vi "sv_UFF58 Get Channel Name.vi"(0 "channel name":string) -> (4 "numerator channel name":string, 6 "denominator channel name":string)   [LabVIEW 2017, in "SoundVib_UFF58.lvlib"]
doc: "This VI extracts <B>numerator channel name</B> and <B>denominator channel name</B> from <B>channel name</B>. It is used mainly when we want to get the channel name from the spectrum info."
uses:
  <vilib>/addons/Sound and Vibration/svt_UFF58/SoundVib_UFF58.lvlib
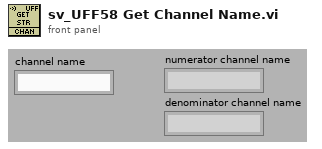
[diagram p1: front panel]
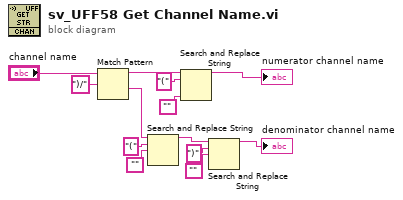
[diagram p0: block diagram]
diagram:
  n1 = Match Pattern(string="channel name", regular expression=")/") -> (before substring=w10:string, after substring=w6:string)  [unwired: 1 in, 2 out]
  n2 = Search and Replace String(input string=w6, search string="(", replace string="") -> (result string=w9:string)  [unwired: 5 in, 3 out]
  n3 = Search and Replace String(input string=w10, search string="(", replace string="") -> (result string=→"numerator channel name":string)  [unwired: 5 in, 3 out]
  n4 = Search and Replace String(input string=w9, search string=")", replace string="") -> (result string=→"denominator channel name":string)  [unwired: 5 in, 3 out]
